vi "Day3.vi"() -> ()   [LabVIEW 2017]
panel:
  in  "Proportional Gain":dbl
  out "Error":dbl
  out "Iterations":i32
  in  "Speed":dbl
  in  "Rotations to do":dbl
  in  "Stop Button":bool
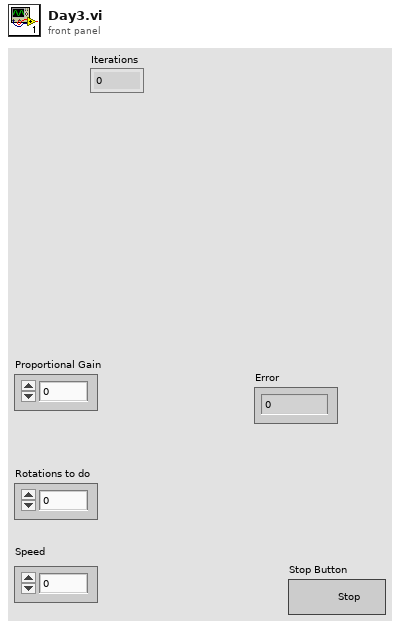
[diagram p1: front panel]
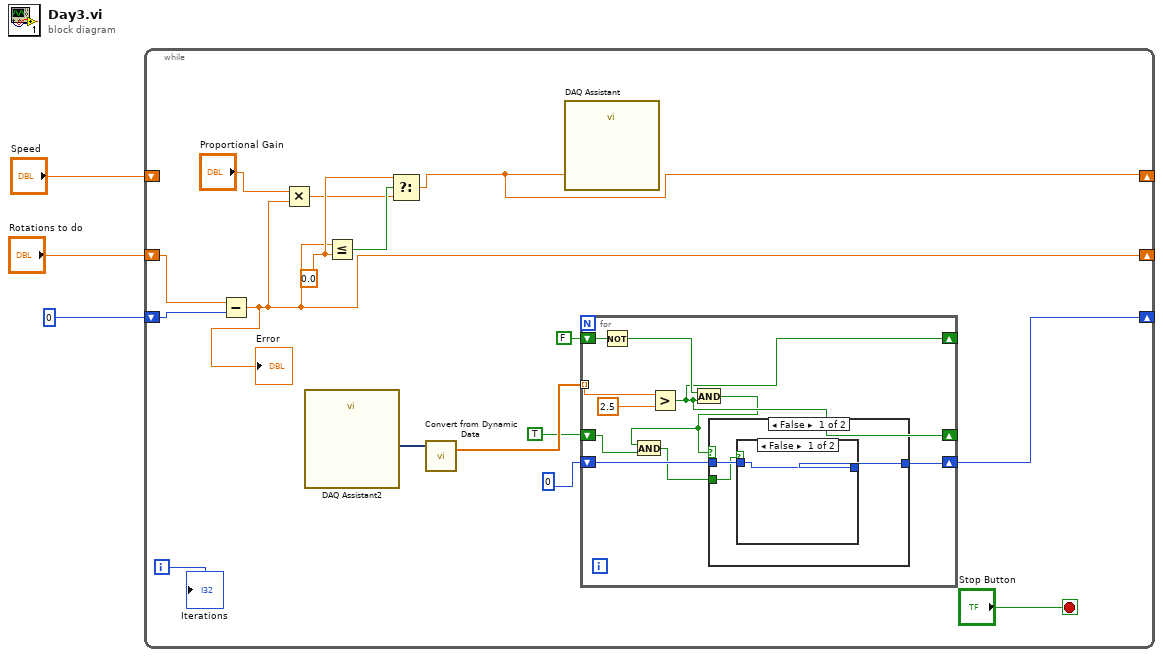
[diagram p0: block diagram]
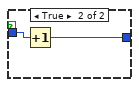
[diagram p2: hidden frame]
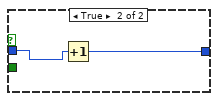
[diagram p3: hidden frame]
diagram:
  n1 = while {
    shift-right: [w13] -> _
    shift-left: "Speed" -> [_]
    shift-right: [w7] -> _
    shift-left: "Rotations to do" -> [w17]
    shift-right: [w9] -> _
    shift-left: 0 -> [w18]
    i -> [w14]
    stop <- "Stop Button" stop-if-true
    w15 = 0.0 ("y")
    n2 = Subtract(x=w17, y=w18) -> (x-y=w7:dbl)
    "Error" <- w7
    n3 = Multiply(x="Proportional Gain", y=w7) -> (x*y=w5:dbl)
    n4 = call "DAQ Assistant2"() -> ("data"=w12:dynamicdata)  [unwired: 17 in, 2 out]
    n5 = Less Or Equal?(x=w7, y=w15) -> (x <= y?=w16:bool)
    n6 = Select(t=w15, s=w16, f=w5) -> (s? t:f=w13:dbl)
    n7 = call "Convert from Dynamic Data"("Dynamic Data Type"=w12) -> ("Array"=w11:dbl[])  [unwired: 3 in]
    n8 = call "DAQ Assistant"("data"=w13) -> ()  [unwired: 17 in, 2 out]
    n9 = for {
      tunnel: w11 -> [w29] mode=indexing
      shift-right: [w23] -> _
      shift-left: FALSE -> [w27]
      shift-right: [w24] -> w9
      shift-left: 0 -> [w25]
      shift-right: [w23] -> _
      shift-left: TRUE -> [w22]
      n10 = Not(x=w27) -> (.not. x?=w26:bool)
      n11 = Greater?(x=w29, y=2.5) -> (0:w23:bool)
      n12 = And(x=w26, y=w23) -> (x .and. y?=w21:bool)
      n13 = And(x=w21, y=w22) -> (x .and. y?=w20:bool)
      n14 = case shown="False" w21 {
        tunnel: w25 -> [w32 w37]
        tunnel: [w31 w36] -> w24
        tunnel: w20 -> [w30 _]
        frame False {
          n15 = case shown="False" w30 {
            tunnel: w32 -> [w33 w34]
            tunnel: [w33 w35] -> w31
            frame False {
            }
            frame True {
              n16 = Increment(x=w34) -> (x+1=w35:i32)
            }
          }
        }
        frame True {
          n17 = Increment(x=w37) -> (x+1=w36:i32)
        }
      }
    }
    "Iterations" <- w14
  }
